vi "数据分类.vi"(4 "样品标记筛选-排除":string[](array[string]), 5 "包含删除？":enum8{"False", "True", "Mixed"}(c332), 6 "样品标记筛选-包含":string[](array[string]), 7 "测试类型":T1, 9 "所有类型":bool, 11 "数组输入":T2[](array[typedef])) -> (0 "数据索引":i32[](array[numeric]), 3 "数组输出":T2[](array[typedef]))   [LabVIEW 2021]
uses:
  <vilib>/regexp/Match Regular Expression.xnode
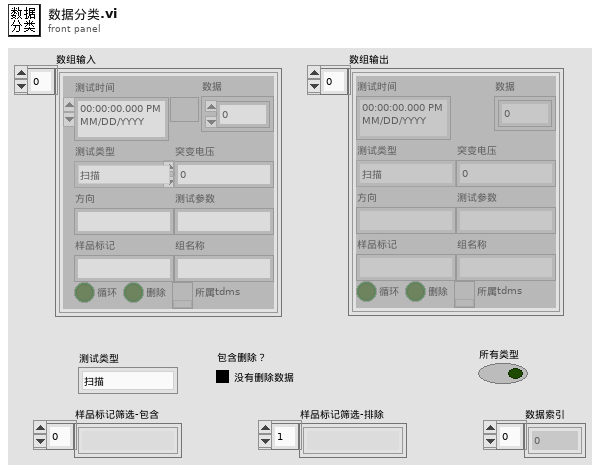
[diagram p1: front panel]
types:
  T1 = typedef "测试类型.ctl" = enum16{"扫描", "脉冲", "维持时间"}
  T2 = typedef "测试数据类型.ctl" = cluster{"测试时间":timestamp, "测试类型":T1, "方向":string, "样品标记":string, "测试参数":string, "循环":bool, "删除":bool, "组名称":string, "所属tdms":refnum<k34>, "突变电压":i32, "数据":dbl[][]}
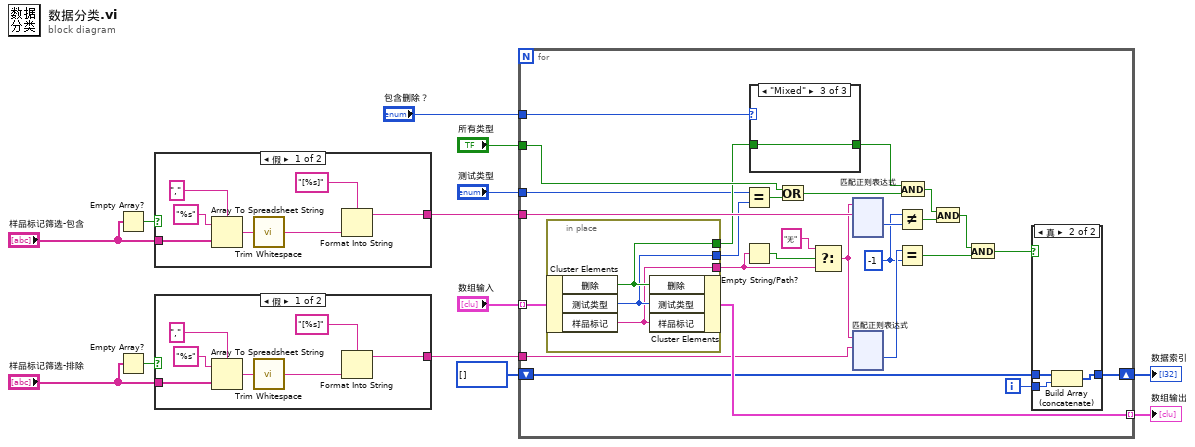
[diagram p0: block diagram]
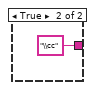
[diagram p2: hidden frame]
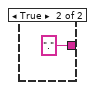
[diagram p3: hidden frame]
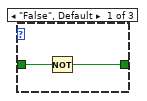
[diagram p4: hidden frame]
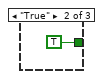
[diagram p5: hidden frame]
diagram:
  n1 = Empty Array?(array="样品标记筛选-包含") -> (empty?=w6:bool)
  n2 = Empty Array?(array="样品标记筛选-排除") -> (empty?=w3:bool)
  n3 = case shown="假" w6 {
    tunnel: "样品标记筛选-包含" -> [w15 _]
    tunnel: [w14 "."] -> w5
    frame False {
      n4 = Array To Spreadsheet String(delimiter (Tab)="," ("分隔符(Tab)"), array=w15, 3:"%s" ("格式字符串")) -> (spreadsheet string=w18:string)
      n5 = call <vilib>:"Trim Whitespace.vi"("string"=w18) -> ("trimmed string"=w20:string)  [unwired: 1 in]
      n6 = Format Into String(format string="[%s]" ("格式字符串"), w20) -> (resulting string=w14:string)  [unwired: 2 in, 1 out]
    }
    frame True {
    }
  }
  n7 = case shown="假" w3 {
    tunnel: "样品标记筛选-排除" -> [w27 _]
    tunnel: [w22 "\\cc"] -> w2
    frame False {
      n8 = Array To Spreadsheet String(delimiter (Tab)="," ("分隔符(Tab)"), array=w27, 3:"%s" ("格式字符串")) -> (spreadsheet string=w25:string)
      n9 = call <vilib>:"Trim Whitespace.vi"("string"=w25) -> ("trimmed string"=w23:string)  [unwired: 1 in]
      n10 = Format Into String(format string="[%s]" ("格式字符串"), w23) -> (resulting string=w22:string)  [unwired: 2 in, 1 out]
    }
    frame True {
    }
  }
  n11 = for {
    tunnel: "数组输入" -> [w56] mode=indexing
    tunnel: [w55] -> w11 mode=indexing
    shift-right: [w52] -> w13
    shift-left: i32[] [] ("扫描") -> [w54]
    tunnel: "测试类型" -> [w31]
    tunnel: "所有类型" -> [w50]
    tunnel: w5 -> [w49]
    tunnel: w2 -> [w48]
    tunnel: "包含删除？" -> [w39]
    i -> [w51]
    w44 = -1 ("y")
    n12 = in-place {
      in-place-border: [w301] -> w38
      in-place-border: [w300] -> w30
      in-place-border: [w299] -> w42
      n13 = in-place-cluster #1(w56) -> ("删除"=w301:bool, "测试类型"=w300:T1, "样品标记"=w299:string)
      n14 = in-place-cluster #1("删除"=w301, "测试类型"=w300, "样品标记"=w299) -> (w55:T2)
    }
    n15 = Equal?(x=w31, y=w30) -> (x = y?=w53:bool)
    n16 = Empty String/Path?(string/path=w42) -> (empty?=w43:bool)
    n17 = case shown="\"Mixed\"" w39 {
      tunnel: w38 -> [w58 _ w60]
      tunnel: [w57 TRUE w60] -> w32
      frame "False", Default {
        n18 = Not(x=w58) -> (.not. x?=w57:bool)
      }
      frame "True" {
      }
      frame "Mixed" {
      }
    }
    n19 = Or(x=w50, y=w53) -> (x .or. y?=w33:bool)
    n20 = Select(t="无", s=w43, f=w42) -> (s? t:f=w40:string)
    n21 = xnode "匹配正则表达式"("输入字符串"=w40, "正则表达式"=w49) -> ("匹配后偏移量"=w45:i32)  [unwired: 4 in, 4 out]
    n22 = xnode "匹配正则表达式"("输入字符串"=w40, "正则表达式"=w48) -> ("匹配后偏移量"=w47:i32)  [unwired: 4 in, 4 out]
    n23 = Not Equal?(x=w44, y=w45) -> (x != y?=w34:bool)
    n24 = Equal?(x=w47, y=w44) -> (x = y?=w36:bool)
    n25 = And(x=w32, y=w33) -> (x .and. y?=w35:bool)
    n26 = And(x=w35, y=w34) -> (x .and. y?=w37:bool)
    n27 = And(x=w37, y=w36) -> (x .and. y?=w46:bool)
    n28 = case shown="真" w46 {
      tunnel: w54 -> [w295 w298]
      tunnel: [w295 w297] -> w52
      tunnel: w51 -> [_ w296]
      frame False {
      }
      frame True {
        n29 = Build Array (concatenate)(w298, w296) -> (w297:i32[])
      }
    }
  }
  "数组输出" <- w11
  "数据索引" <- w13
